vi "Configure Trigger.vi"(6 "Manual Trigger Delay (0.0 s)":dbl format="%.5g", 8 "error in (no error)":errorcluster, 9 "Auto Delay (T: Enable)":bool=TRUE, 10 "Trigger Source (0: Immediate)":u16(ring) items=["Immediate", "Software (Bus)", "External"], 11 "VISA resource name":refnum<visa-resource-name>) -> (0 "error out":errorcluster, 3 "VISA resource name out":refnum<visa-resource-name>)   [LabVIEW 2014, in "Fluke 884X Series.lvlib"]
doc: "Configures the trigger settings on the instrument.\n\n<B>Note:</B>\n\nThis VI will only be used with the low level Data VIs, as the high level VIs already contain this functionality."
uses:
  Fluke 884X Series.lvlib
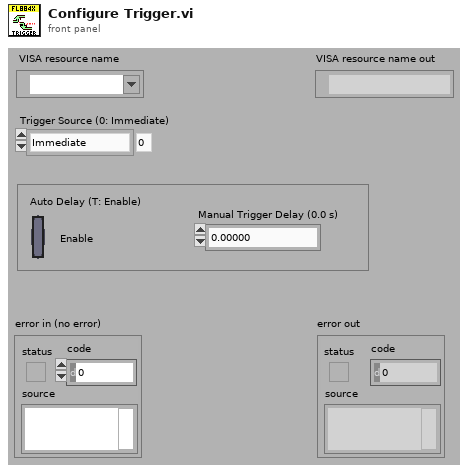
[diagram p1: front panel]
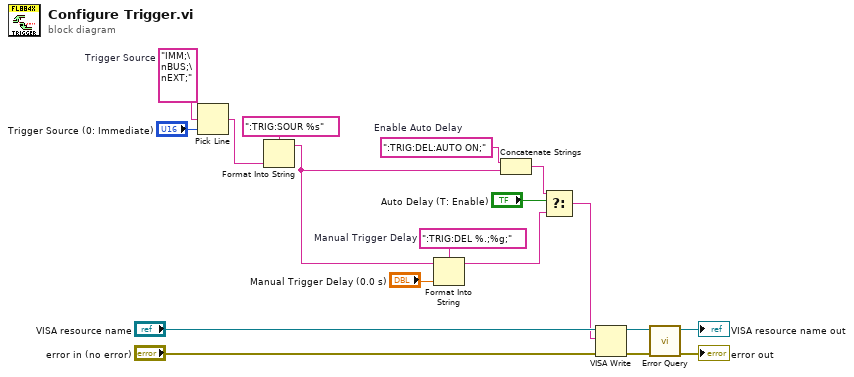
[diagram p0: block diagram]
diagram:
  w2 = ":TRIG:DEL:AUTO ON;"  # Enable Auto Delay
  w12 = ":TRIG:DEL %.;%g;"  # Manual Trigger Delay
  w16 = "IMM;\nBUS;\nEXT;"  # Trigger Source
  n1 = Pick Line(multi-line string=w16, line index="Trigger Source (0: Immediate)") -> (output string=w8:string)  [unwired: 1 in]
  n2 = Format Into String(format string=":TRIG:SOUR %s", w8) -> (resulting string=w1:string)  [unwired: 2 in, 1 out]
  n3 = Format Into String(format string=w12, initial string=w1, "Manual Trigger Delay (0.0 s)") -> (resulting string=w5:string)  [unwired: 1 in, 1 out]
  n4 = Concatenate Strings(w2, w1) -> (w3:string)
  n5 = Select(t=w3, s="Auto Delay (T: Enable)", f=w5) -> (s? t:f=w4:string)
  n6 = VISA Write(VISA resource name="VISA resource name", write buffer=w4, error in (no error)="error in (no error)") -> (VISA resource name out=w15:refnum<visa-resource-name>, error out=w14:errorcluster)  [unwired: 1 out]
  n7 = call "Error Query.vi"("error in (no error)"=w14, "VISA resource name"=w15) -> ("error out"=→"error out":errorcluster, "VISA resource name out"=→"VISA resource name out":refnum<visa-resource-name>)  [unwired: 6 in, 2 out]
